vi "DAQ - WRITE - Simple digital signal.vi"(8 "error in":errorcluster, 11 "Digital Output Channel":tag="Dev1/ao0") -> (0 "error out":errorcluster, 3 "task out":refnum<k21>)   [LabVIEW 2017]
uses:
  <vilib>/DAQmx/create/channels.llb/DAQmx Create Channel (DO-Digital Output).vi
  <resource>/objmgr/daqmx.rc
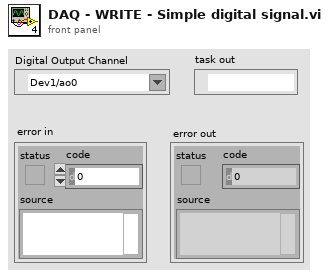
[diagram p1: front panel]
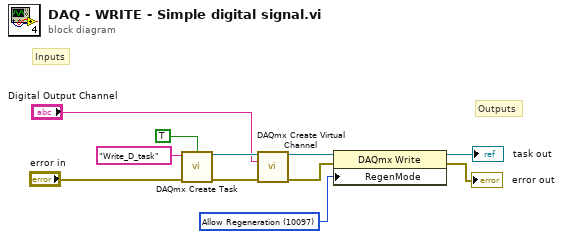
[diagram p0: block diagram]
diagram:
  w1 = 10097 items=["Allow Regeneration"=10097, "Do Not Allow Regeneration"=10158] ("RegenMode")
  # "Inputs"
  # "Outputs"
  n1 = call <vilib>:"DAQmx Create Task.vi"("new task name"="Write_D_task", "auto cleanup"=TRUE, "error in"="error in") -> ("task out"=w8:refnum<k21>, "error out"=w9:errorcluster)  [unwired: 11 in]
  n2 = call-poly <vilib>:"DAQmx Create Virtual Channel.vi"("task in"=w8, "lines"="Digital Output Channel", "error in"=w9) -> ("task out"=w5:refnum<k21>, "error out"=w2:errorcluster)  [unwired: 11 in]
  n3 = property class="DAQmx Write"(reference=w5, error in=w2, "RegenMode"=w1) -> (reference out=→"task out":refnum<k21>, error out=→"error out":errorcluster)
